vi "deque.vi"(4 "timeout":dbl=1.0, 6 "que_out?":bool=TRUE, 8 "error in (no error)":errorcluster, 11 "py in":T1) -> (0 "error out":errorcluster, 1 "value":string, 2 "response":T3, 3 "py out":T1)   [LabVIEW 2022 SP3, in "pythonq.lvlib"]
uses:
  pythonq.lvlib
  py_result.ctl
  py_session.ctl
  py_cluster.ctl
panel:
  out "raw":string
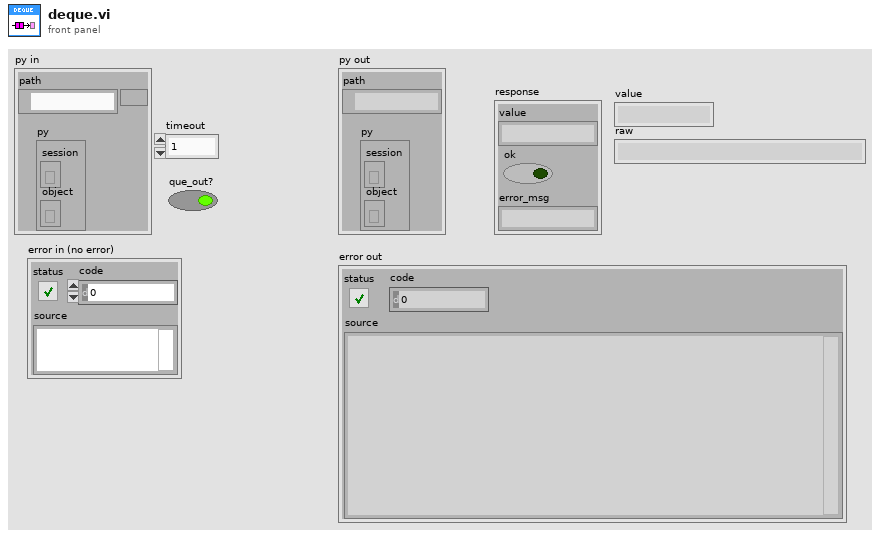
[diagram p1: front panel]
types:
  T1 = typedef "pythonq.lvlib/py_cluster.ctl" = cluster{"path":path, "py":T2}
  T2 = typedef "pythonq.lvlib/py_session.ctl" = cluster{"session":refnum<k35>, "object":refnum<k38>}
  T3 = typedef "pythonq.lvlib/py_result.ctl" = cluster{"value":string, "ok":bool, "error_msg":string}
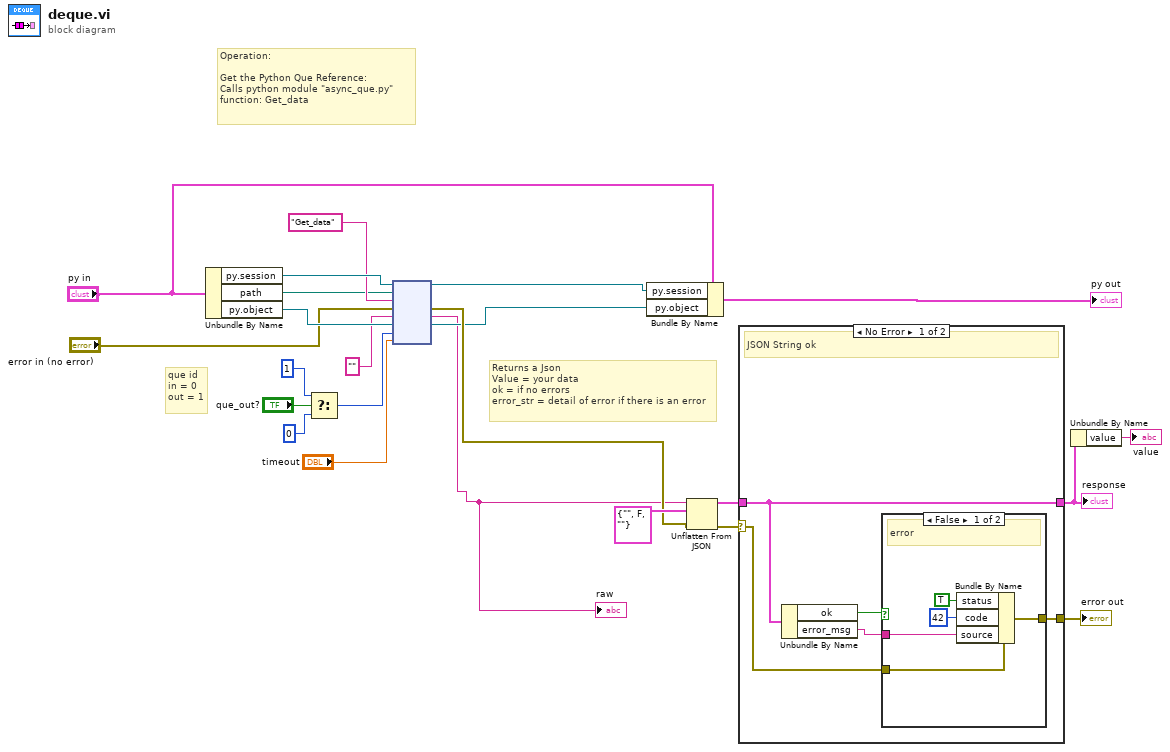
[diagram p0: block diagram]
diagram:
  # "Returns a Json\nValue = your data\nok = if no errors\nerror_str = detail of error if there is an error"
  # "que id\nin = 0\nout = 1"
  # "Operation:\n\nGet the Python Que Reference:\nCalls python module \"async_que.py\"\nfunction: Get_data"
  n1 = Unbundle By Name("py in") -> ("py.session"=w22:refnum<k35>, "path"=w9:path, "py.object"=w23:refnum<k38>)
  n2 = Select(t=1, s="que_out?", f=0) -> (s? t:f=w3:i32)
  n3 = node(w22, w9, "Get_data" ("function name"), "error in (no error)", "", w23, w3, "timeout") -> (w14:refnum<k35>, w18:errorcluster, w1:string, w13:refnum<k38>)  [unwired: 2 in, 2 out]
  "raw" <- w1
  n4 = Bundle By Name(cluster="py in", "py.session"=w14, "py.object"=w13) -> (→"py out":T1)
  n5 = Unflatten From JSON(JSON string=w1, type and defaults=T3 {"value"="", "ok"=FALSE, "error_msg"=""}, error in (no error)=w18) -> (value=w17:T3, error out=w16:errorcluster)  [unwired: 4 in]
  n6 = case shown="No Error" w16 {
    selector: w16 -> [w26 w35]
    tunnel: w17 -> [w28 w36]
    tunnel: [w28 w36] -> w12
    tunnel: [w25 w35] -> w15
    frame No Error {
      # "JSON String ok"
      n7 = Unbundle By Name(w28) -> ("ok"=w27:bool, "error_msg"=w24:string)
      n8 = case shown="False" w27 {
        tunnel: w26 -> [w33 w34]
        tunnel: [w31 w34] -> w25
        tunnel: w24 -> [w30 _]
        frame False {
          # "error"
          n9 = Bundle By Name(cluster=w33, "status"=TRUE, "code"=42, "source"=w30) -> (w31:errorcluster)
        }
        frame True {
          # "no error"
        }
      }
    }
    frame Error {
    }
  }
  "error out" <- w15
  "response" <- w12
  n10 = Unbundle By Name(w12) -> ("value"=→"value":string)
